vi "plant_pause.vi"(0 "Dataflow In":errorcluster, 1 "Pause":refnum<vi>) -> (5 "Dataflow Out":errorcluster)   [LabVIEW 2019]
uses:
  lib/libSimulationControl/libSimulationControl.lvlib
panel:
  # "*******************************************************************\nBiogas Plant Control\n\nAuthor: Paul Zügel\nGCSC-Frankfurt am Main 2020\n\n*******************************************************************"
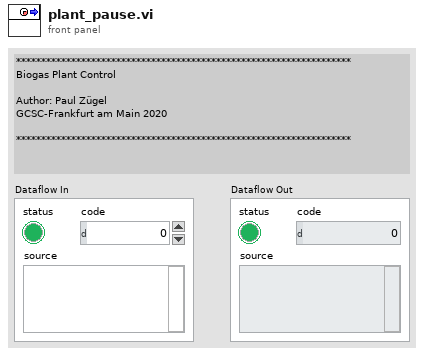
[diagram p1: front panel]
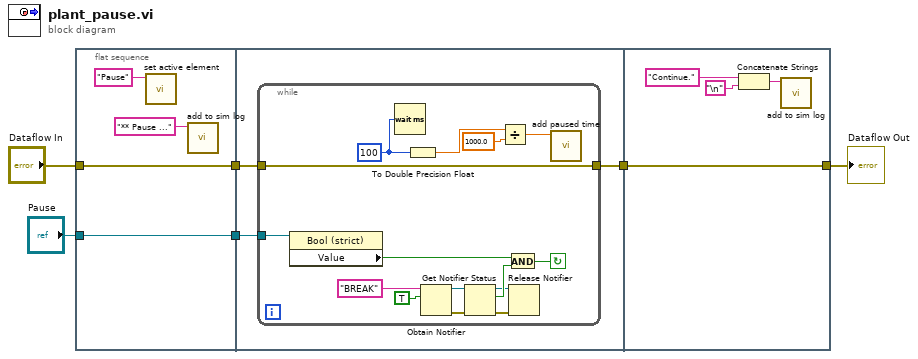
[diagram p0: block diagram]
diagram:
  n1 = flat-sequence {
    tunnel: "Pause" -> [w9]
    tunnel: "Dataflow In" -> [w10]
    tunnel: [w10] -> w5
    tunnel: [w9] -> w4
    tunnel: w5 -> [w13]
    tunnel: w4 -> [w11]
    tunnel: [w12] -> w3
    tunnel: [w32] -> w1
    tunnel: w3 -> [w32]
    frame #0 {
      n2 = call "set active element.vi"("elem"="Pause") -> ()  [unwired: 10 in, 1 out]
      n3 = call "add to sim log.vi"("log"="** Pause ..." ("string")) -> ()  [unwired: 10 in, 1 out]
    }
    frame #1 {
      n4 = while {
        tunnel: w13 -> [w28]
        tunnel: [w28] -> w12
        tunnel: w11 -> [w27]
        stop <- w20 continue-if-true
        w19 = u32 100 ("milliseconds to wait")
        n5 = property class="Bool (strict)"(reference=w27) -> ("Value"=w22:bool)  [unwired: 1 in, 2 out]
        n6 = Wait (ms)(milliseconds to wait=w19) -> ()  [unwired: 1 out]
        n7 = To Double Precision Float(number=w19) -> (double precision float=w17:dbl)
        n8 = Obtain Notifier(name (unnamed)="BREAK", notification data type=TRUE) -> (notifier out=w24:refnum<notifier>, error out=w23:errorcluster)  [unwired: 2 in, 1 out]
        n9 = Get Notifier Status(notifier=w24, error in (no error)=w23) -> (notifier out=w15:refnum<notifier>, current notification=w21:bool, error out=w14:errorcluster)  [unwired: 2 out]
        n10 = Divide(x=w17, y=1000.0) -> (x/y=w16:dbl)
        n11 = And(x=w22, y=w21) -> (x .and. y?=w20:bool)
        n12 = Release Notifier(notifier=w15, error in (no error)=w14) -> ()  [unwired: 1 in, 3 out]
        n13 = call "add paused time.vi"("time"=w16) -> ()  [unwired: 10 in, 1 out]
      }
    }
    frame #2 {
      n14 = Concatenate Strings("Continue." ("string"), "\n") -> (w29:string)
      n15 = call "add to sim log.vi"("log"=w29) -> ()  [unwired: 10 in, 1 out]
    }
  }
  "Dataflow Out" <- w1
